vi "Drive Direction.vi"(6 "Drive Dev Ref":T1={"DeviceStatus"={"status"=FALSE, "code"=0, "source"=""}, "Type"=enum."PWM", "PWM"={"PWM Channel"=enum."Invalid", "DeadBand"={"Name"="", "maxPositivePwm"=0, "minPositivePwm"=0, "centerPwm"=0, "maxNegativePwm"=0, "minNegativePwm"=0, "angularRange"=0}}, "CAN"={"Device Number"=0, "SetOutput VI Ref"=variant(refnum<vi> refnum), "GetOutput VI Ref"=variant(refnum<vi> refnum), "Enable VI Ref"=variant(refnum<vi> refnum), "Disable VI Ref"=variant(refnum<vi> refnum), "Data"=variant}, "Invert"=FALSE}, 7 "Swerve Dev Ref":T1={"DeviceStatus"={"status"=FALSE, "code"=0, "source"=""}, "Type"=enum."PWM", "PWM"={"PWM Channel"=enum."Invalid", "DeadBand"={"Name"="", "maxPositivePwm"=0, "minPositivePwm"=0, "centerPwm"=0, "maxNegativePwm"=0, "minNegativePwm"=0, "angularRange"=0}}, "CAN"={"Device Number"=0, "SetOutput VI Ref"=variant(refnum<vi> refnum), "GetOutput VI Ref"=variant(refnum<vi> refnum), "Enable VI Ref"=variant(refnum<vi> refnum), "Disable VI Ref"=variant(refnum<vi> refnum), "Data"=variant}, "Invert"=FALSE}, 8 "Module Number":i32, 10 "Wheel Power":dbl format="%#_13g", 11 "Desired direction (radians)":dbl=6.283185307179586 format="%#_13g") -> ()   [LabVIEW 2016]
uses:
  <vilib>/Rock Robotics/WPI/MotorControl/WPI_MotorControlDeviceRef.ctl
  <vilib>/Rock Robotics/WPI/MotorControl/WPI_MotorControlType.ctl
  <vilib>/Rock Robotics/SystemInterfaces/DIO/FPGA_DIOPWMChannel.ctl
  <vilib>/Rock Robotics/WPI/PWM/WPI_PWMDeadband.ctl
  Main/Robot Global Data.vi
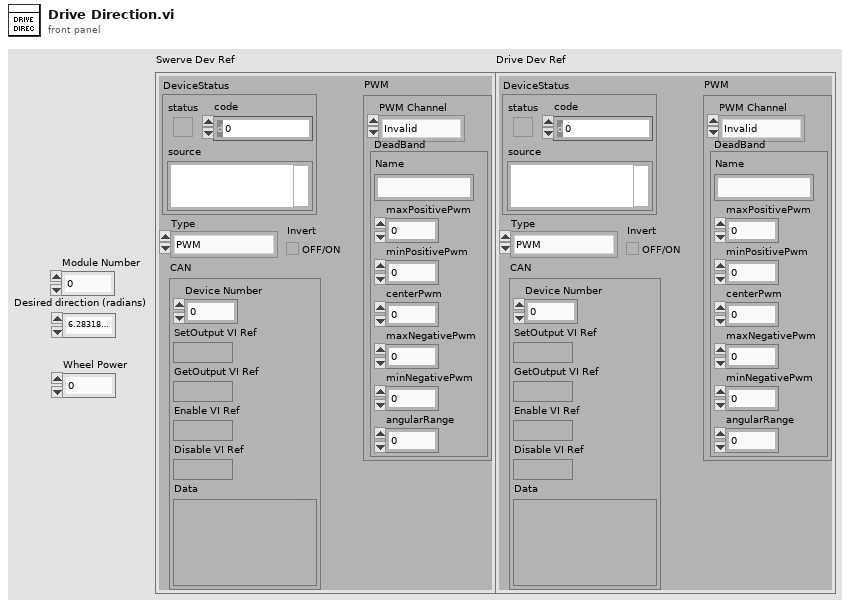
[diagram p1: front panel]
types:
  T1 = typedef "WPI_MotorControlDeviceRef.ctl" = cluster{"DeviceStatus":errorcluster, "Type":T2, "PWM":cluster{"PWM Channel":T3, "DeadBand":T4}, "CAN":cluster{"Device Number":u8, "SetOutput VI Ref":variant, "GetOutput VI Ref":variant, "Enable VI Ref":variant, "Disable VI Ref":variant, "Data":variant}, "Invert":bool}
  T2 = typedef "WPI_MotorControlType.ctl" = enum16{"PWM", "CAN"}
  T3 = typedef "FPGA_DIOPWMChannel.ctl" = enum8{"PWM 0", "PWM 1", "PWM 2", "PWM 3", "PWM 4", "PWM 5", "PWM 6", "PWM 7", "PWM 8", "PWM 9", "PWM MXP 0", "PWM MXP 1", "PWM MXP 2", "PWM MXP 3", "PWM MXP 4", "PWM MXP 5", "PWM MXP 6", "PWM MXP 7", "PWM MXP 8", "PWM MXP 9", "Invalid"}
  T4 = typedef "WPI_PWMDeadband.ctl" = cluster{"Name":string, "maxPositivePwm":i32, "minPositivePwm":i32, "centerPwm":i32, "maxNegativePwm":i32, "minNegativePwm":i32, "angularRange":u16}
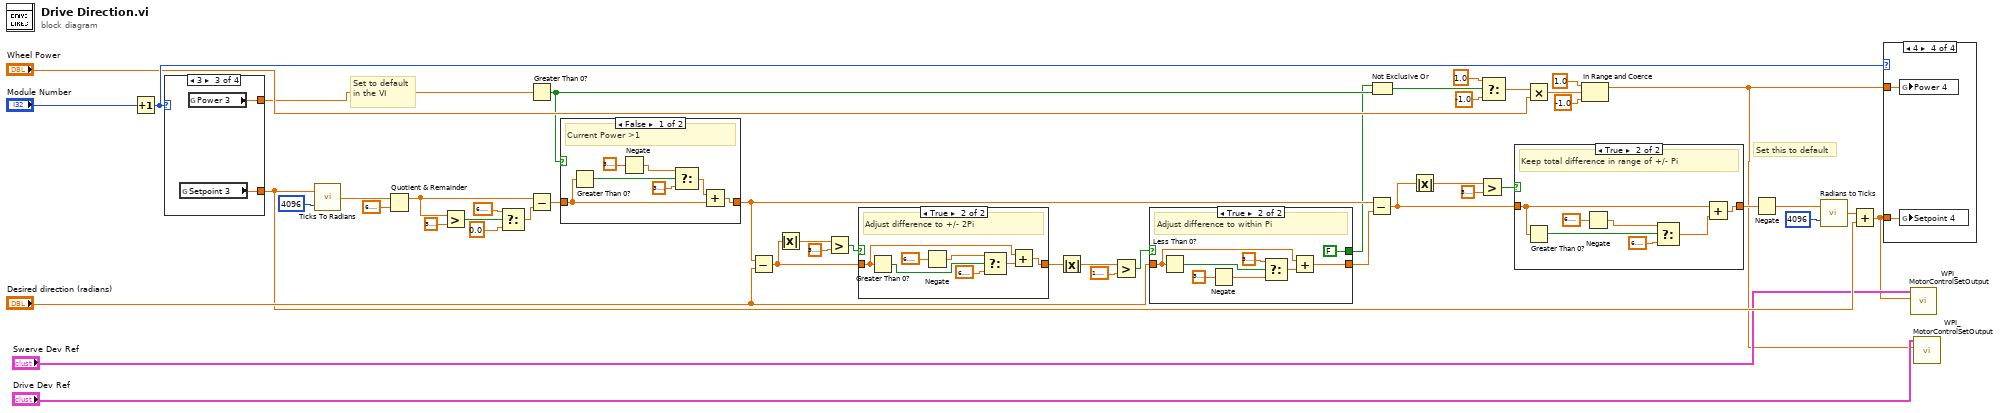
[diagram p0: block diagram]
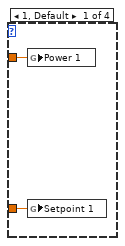
[diagram p2: hidden frame]
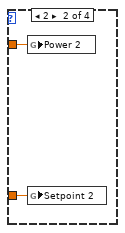
[diagram p3: hidden frame]
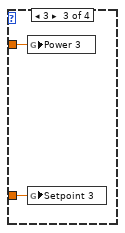
[diagram p4: hidden frame]
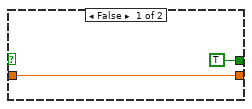
[diagram p6: hidden frame]
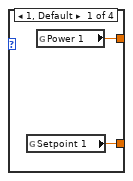
[diagram p9: hidden frame]
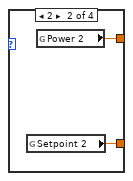
[diagram p10: hidden frame]
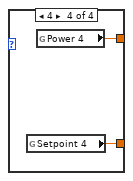
[diagram p11: hidden frame]
diagram:
  # "Set this to default"
  # "Set to default\nin the VI"
  n1 = Increment(x="Module Number") -> (x+1=w17:i32)
  n2 = case shown="3" w17 {
    tunnel: [w48 w51 w52 w55] -> w5
    tunnel: [w49 w50 w53 w54] -> w6
    frame 1, Default {
      n3 = global read "Robot Global Data.vi" "Setpoint 1"() -> (w48:dbl)
      n4 = global read "Robot Global Data.vi" "Power 1"() -> (w49:dbl)
    }
    frame 2 {
      n5 = global read "Robot Global Data.vi" "Setpoint 2"() -> (w51:dbl)
      n6 = global read "Robot Global Data.vi" "Power 2"() -> (w50:dbl)
    }
    frame 3 {
      n7 = global read "Robot Global Data.vi" "Setpoint 3"() -> (w52:dbl)
      n8 = global read "Robot Global Data.vi" "Power 3"() -> (w53:dbl)
    }
    frame 4 {
      n9 = global read "Robot Global Data.vi" "Setpoint 4"() -> (w55:dbl)
      n10 = global read "Robot Global Data.vi" "Power 4"() -> (w54:dbl)
    }
  }
  n11 = call "Ticks To Radians.vi"("Ticks/Rev"=4096, "Ticks"=w5) -> ("Radians"=w39:dbl)
  n12 = Quotient & Remainder(x=w39, y=6.283185307179586) -> (x-y*floor(x/y)=w37:dbl)  [unwired: 1 out]
  n13 = Greater?(x=w37, y=3.141592653589793) -> (0:w43:bool)
  n14 = Select(t=6.283185307179586, s=w43, f=0.0) -> (s? t:f=w40:dbl)
  n15 = Greater Than 0?(x=w6) -> (x > 0?=w8:bool)
  n16 = Subtract(x=w37, y=w40) -> (x-y=w38:dbl)
  n17 = case shown="False" w8 {
    tunnel: w38 -> [w57 w63]
    tunnel: [w56 w63] -> w21
    frame False {
      # "Current Power >1"
      n18 = Greater Than 0?(x=w57) -> (x > 0?=w62:bool)
      n19 = Negate(x=3.141592653589793) -> (-x=w61:dbl)
      n20 = Select(t=w61, s=w62, f=3.141592653589793) -> (s? t:f=w58:dbl)
      n21 = Add(x=w58, y=w57) -> (x+y=w56:dbl)
    }
    frame True {
      # "Current Power >1"
    }
  }
  n22 = Subtract(x=w21, y="Desired direction (radians)") -> (x-y=w33:dbl)
  n23 = Absolute Value(x=w33) -> (abs(x)=w34:dbl)
  n24 = Greater?(x=w34, y=3.141592653589793) -> (0:w36:bool)
  n25 = case shown="True" w36 {
    tunnel: w33 -> [w64 w66]
    tunnel: [w64 w65] -> w30
    frame False {
    }
    frame True {
      # "Adjust difference to +/- 2Pi"
      n26 = Greater Than 0?(x=w66) -> (x > 0?=w71:bool)
      n27 = Negate(x=6.283185307179586) -> (-x=w68:dbl)
      n28 = Select(t=w68, s=w71, f=6.283185307179586) -> (s? t:f=w67:dbl)
      n29 = Add(x=w66, y=w67) -> (x+y=w65:dbl)
    }
  }
  n30 = Absolute Value(x=w30) -> (abs(x)=w31:dbl)
  n31 = Greater?(x=w31, y=1.5707963267948966) -> (0:w29:bool)
  n32 = case shown="True" w29 {
    tunnel: "Desired direction (radians)" -> [w73 w76]
    tunnel: [w73 w75] -> w22
    tunnel: [TRUE FALSE] -> w7
    frame False {
    }
    frame True {
      # "Adjust difference to within Pi"
      n33 = Less Than 0?(x=w76) -> (x < 0?=w81:bool)
      n34 = Negate(x=3.141592653589793) -> (-x=w78:dbl)
      n35 = Select(t=3.141592653589793, s=w81, f=w78) -> (s? t:f=w77:dbl)
      n36 = Add(x=w76, y=w77) -> (x+y=w75:dbl)
    }
  }
  n37 = Subtract(x=w21, y=w22) -> (x-y=w24:dbl)
  n38 = Not Exclusive Or(1:w8, 2:w7) -> (0:w16:bool)
  n39 = Absolute Value(x=w24) -> (abs(x)=w27:dbl)
  n40 = Greater?(x=w27, y=3.141592653589793) -> (0:w26:bool)
  n41 = Select(t=1.0, s=w16, f=-1.0 ("t")) -> (s? t:f=w13:dbl)
  n42 = case shown="True" w26 {
    tunnel: w24 -> [w82 w84]
    tunnel: [w82 w83] -> w23
    frame False {
    }
    frame True {
      # "Keep total difference in range of +/- Pi"
      n43 = Greater Than 0?(x=w84) -> (x > 0?=w89:bool)
      n44 = Negate(x=6.283185307179586) -> (-x=w87:dbl)
      n45 = Select(t=w87, s=w89, f=6.283185307179586) -> (s? t:f=w86:dbl)
      n46 = Add(x=w84, y=w86) -> (x+y=w83:dbl)
    }
  }
  n47 = Multiply(x=w13, y="Wheel Power") -> (x*y=w9:dbl)
  n48 = In Range and Coerce(upper limit=1.0, x=w9, lower limit=-1.0) -> (coerced(x)=w2:dbl)  [unwired: 1 out]
  n49 = Negate(x=w23) -> (-x=w20:dbl)
  n50 = call "Radians to Ticks.vi"("Ticks/rev"=4096, "Radians"=w20) -> ("Ticks"=w18:dbl)
  n51 = Add(x=w18, y=w5) -> (x+y=w1:dbl)
  n52 = case shown="4" w17 {
    tunnel: w1 -> [w91 w93 w95 w97]
    tunnel: w2 -> [w90 w92 w94 w96]
    frame 1, Default {
      n53 = global write "Robot Global Data.vi" "Power 1"(w90) -> ()
      n54 = global write "Robot Global Data.vi" "Setpoint 1"(w91) -> ()
    }
    frame 2 {
      n55 = global write "Robot Global Data.vi" "Power 2"(w92) -> ()
      n56 = global write "Robot Global Data.vi" "Setpoint 2"(w93) -> ()
    }
    frame 3 {
      n57 = global write "Robot Global Data.vi" "Power 3"(w94) -> ()
      n58 = global write "Robot Global Data.vi" "Setpoint 3"(w95) -> ()
    }
    frame 4 {
      n59 = global write "Robot Global Data.vi" "Power 4"(w96) -> ()
      n60 = global write "Robot Global Data.vi" "Setpoint 4"(w97) -> ()
    }
  }
  n61 = call <vilib>:"WPI_MotorControlSetOutput.vi"("Output"=w1, "MotorControlDevRef"="Swerve Dev Ref") -> ()  [unwired: 7 in, 3 out]
  n62 = call <vilib>:"WPI_MotorControlSetOutput.vi"("Output"=w2, "MotorControlDevRef"="Drive Dev Ref") -> ()  [unwired: 7 in, 3 out]
